vi "MS SQL_InRFID_STN10.vi"(4 "RFID":string, 5 "OP10_CRIMP":T1, 8 "error in (no error)":errorcluster, 10 "Serial No":i32, 11 "Ref in":T2={"MS SQL Connection"=refnum, "UDL File"=path "", "Time"="", "DCODE"="", "WIP+1"=0, "MC No?"=0, "POKAYOKE?"=FALSE, "Expected Result"="", "Result [Status]"="", "Clock"=0.0, "RFID"="", "WIP Queue"=refnum, "TS Parameter"={"ProfitCenterCode"="", "LineCode"="", "WorkOrderNumber"="", "Model"="", "Model_with_Prefix"="", "VendorCode"="", "SetParameterDateCode"="", "PokaYoke"=0, "Target"=1, "Live_DateCode"="", "CustomerPartNumber"="", "Hand"="", "sBarcode"=FALSE, "FCA"=0, "Ent_Stamp"=timestamp(0 s since 1904-01-01), "STS_CD"=0.0}, "Data_Queue"=[], "RFID Serial No."=""} {"TS Parameter"."FCA" format="%01d"; "TS Parameter"."Target" min=1 max=100000; "TS Parameter"."PokaYoke" min=0 max=1}) -> (0 "error out":errorcluster, 3 "Ref Out":T2={"MS SQL Connection"=refnum, "UDL File"=path "", "Time"="", "DCODE"="", "WIP+1"=0, "MC No?"=0, "POKAYOKE?"=FALSE, "Expected Result"="", "Result [Status]"="", "Clock"=0.0, "RFID"="", "WIP Queue"=refnum, "TS Parameter"={"ProfitCenterCode"="", "LineCode"="", "WorkOrderNumber"="", "Model"="", "Model_with_Prefix"="", "VendorCode"="", "SetParameterDateCode"="", "PokaYoke"=0, "Target"=1, "Live_DateCode"="", "CustomerPartNumber"="", "Hand"="", "sBarcode"=FALSE, "FCA"=0, "Ent_Stamp"=timestamp(0 s since 1904-01-01), "STS_CD"=0.0}, "Data_Queue"=[], "RFID Serial No."=""} {"TS Parameter"."FCA" format="%01d"; "TS Parameter"."Target" min=1 max=100000; "TS Parameter"."PokaYoke" min=0 max=1})   [LabVIEW 2020]
uses:
  Controls/TD SQL.ctl
  <vilib>/addons/database/Connection.llb/Conn ObjectReference.ctl
  Controls/WIP_State.ctl
  Controls/TS_Parameter.ctl
  <vilib>/addons/database/NI_Database_API.lvlib
panel:
  in  "[CT]":dbl
  in  "[STATUS]":i32
  out "resulting string":string
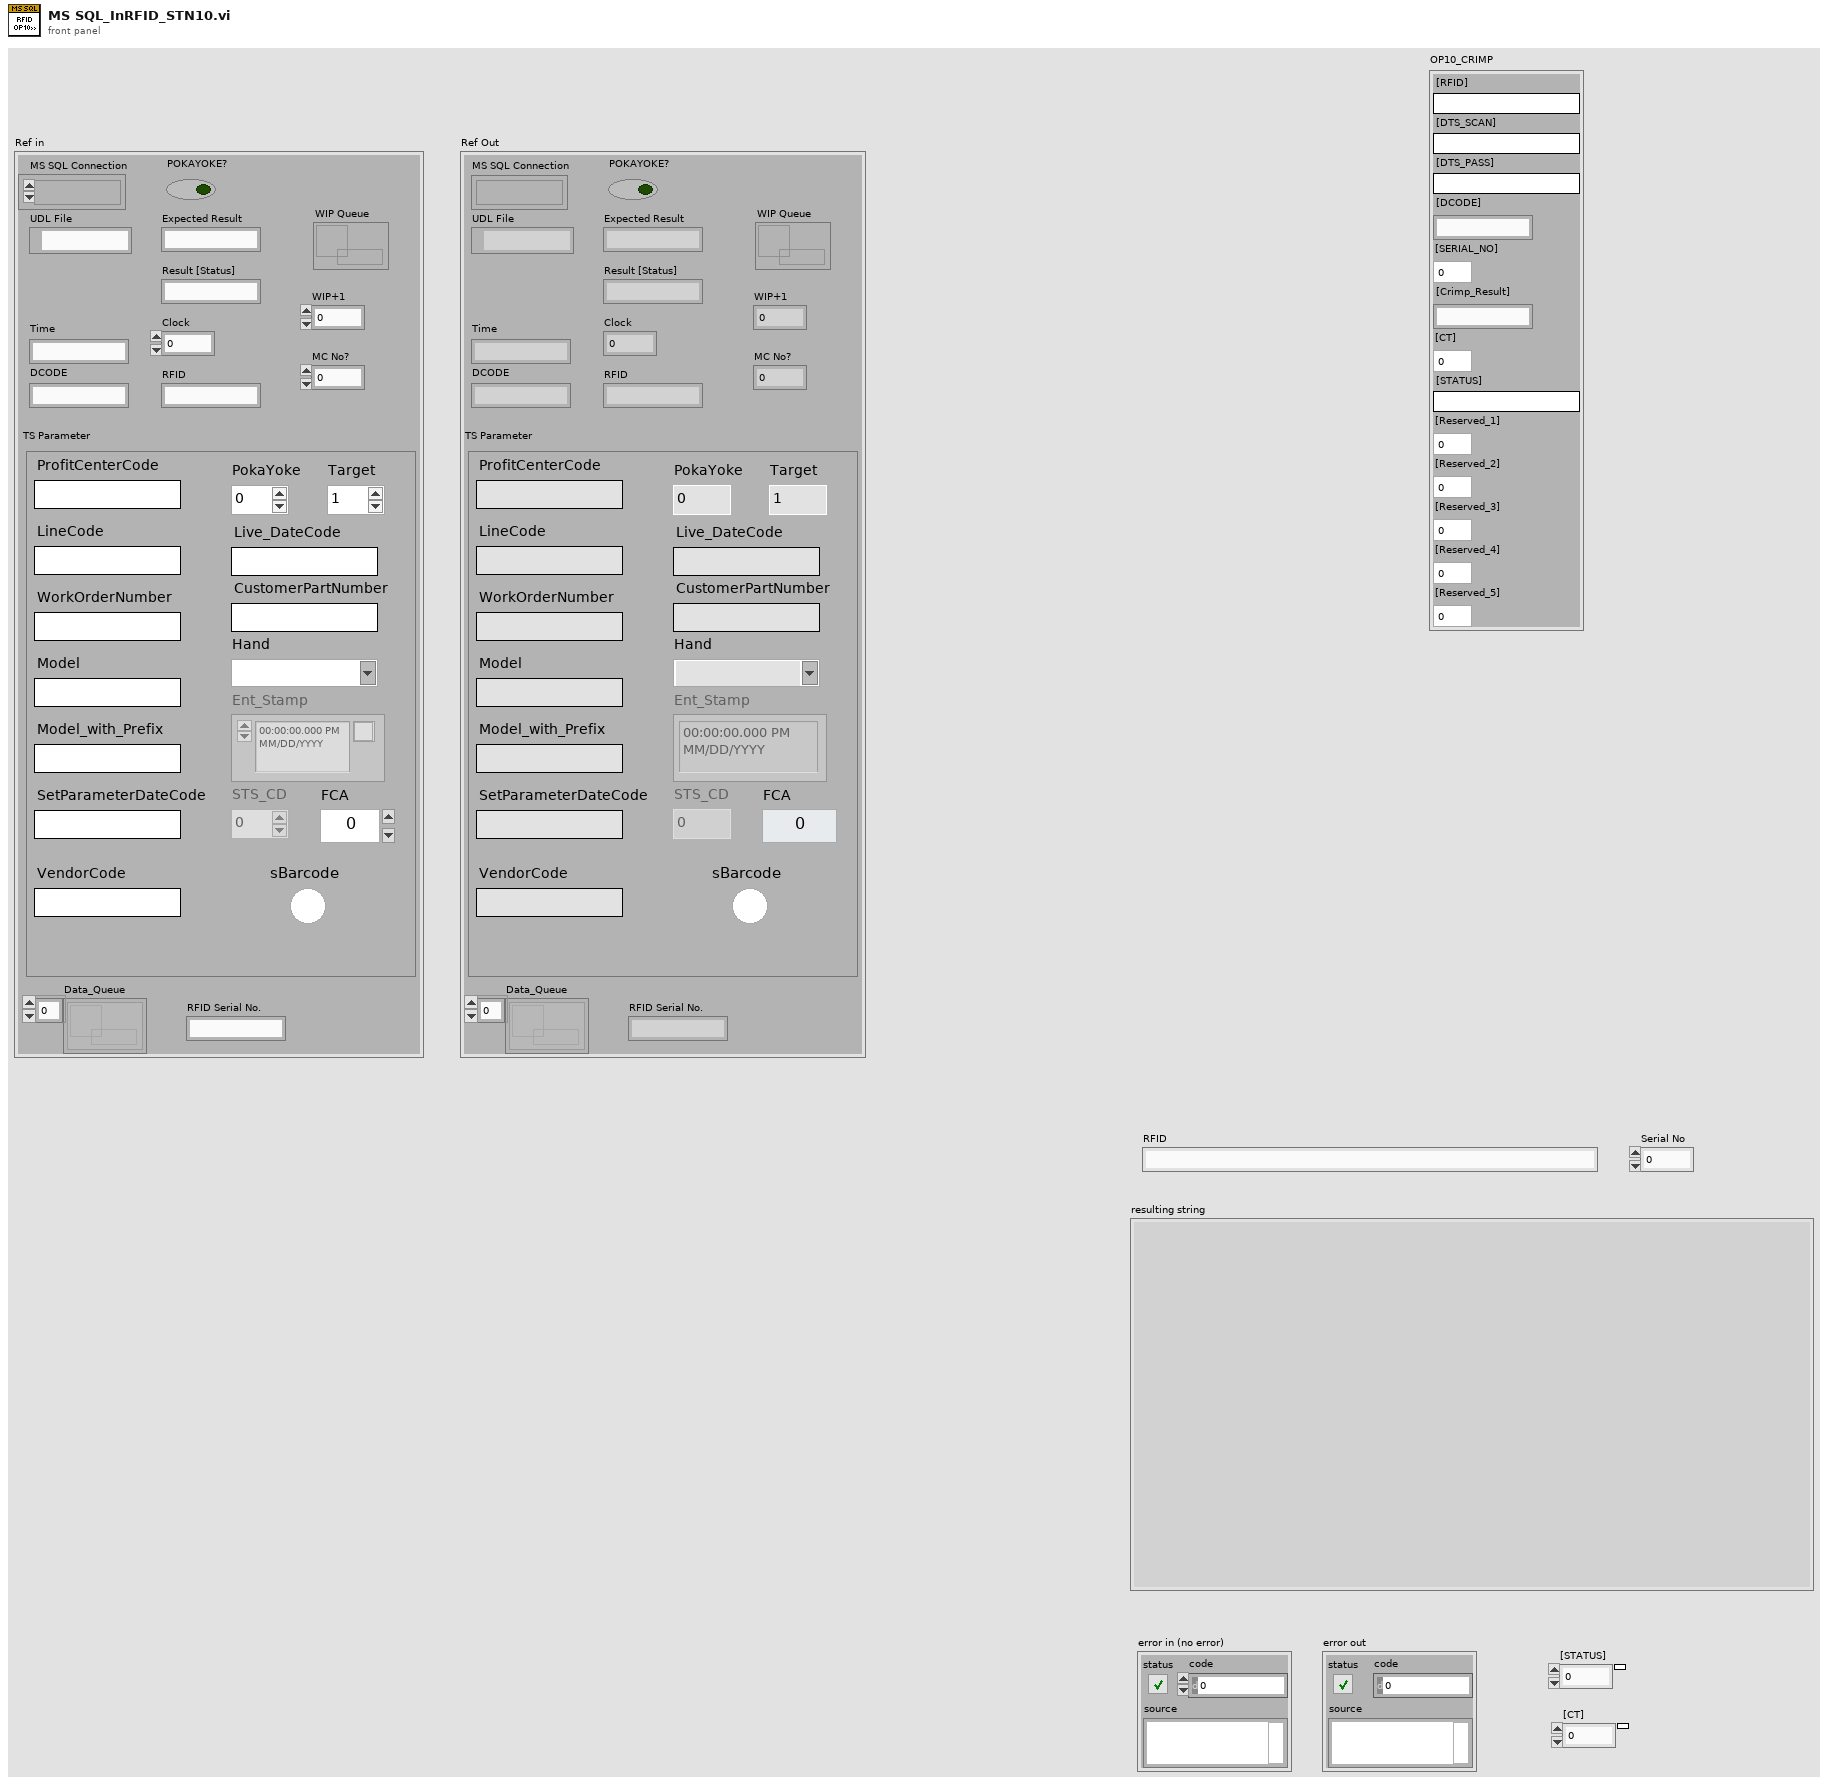
[diagram p1: front panel]
types:
  T1 = cluster{"[RFID]":string, "[DTS_SCAN]":string, "[DTS_PASS]":string, "[DCODE]":string, "[SERIAL_NO]":i32, "[Crimp_Result]":string, "[CT]":dbl, "[STATUS]":string, "[Reserved_1]":dbl, "[Reserved_2]":dbl, "[Reserved_3]":dbl, "[Reserved_4]":dbl, "[Reserved_5]":dbl}
  T2 = typedef "TD SQL.ctl" = cluster{"MS SQL Connection":T3, "UDL File":path, "Time":string, "DCODE":string, "WIP+1":i64, "MC No?":i32, "POKAYOKE?":bool, "Expected Result":string, "Result [Status]":string, "Clock":dbl, "RFID":string, "WIP Queue":refnum<queue>, "TS Parameter":T4, "Data_Queue":refnum<queue>[], "RFID Serial No.":string}
  T3 = typedef "NI_Database_API.lvlib/Conn ObjectReference.ctl" = refnum<k1>
  T4 = typedef "TS_Parameter.ctl" = cluster{"ProfitCenterCode":string, "LineCode":string, "WorkOrderNumber":string, "Model":string, "Model_with_Prefix":string, "VendorCode":string, "SetParameterDateCode":string, "PokaYoke":i32, "Target":i32, "Live_DateCode":string, "CustomerPartNumber":string, "Hand":string, "sBarcode":bool, "FCA":i32, "Ent_Stamp":timestamp, "STS_CD":dbl}
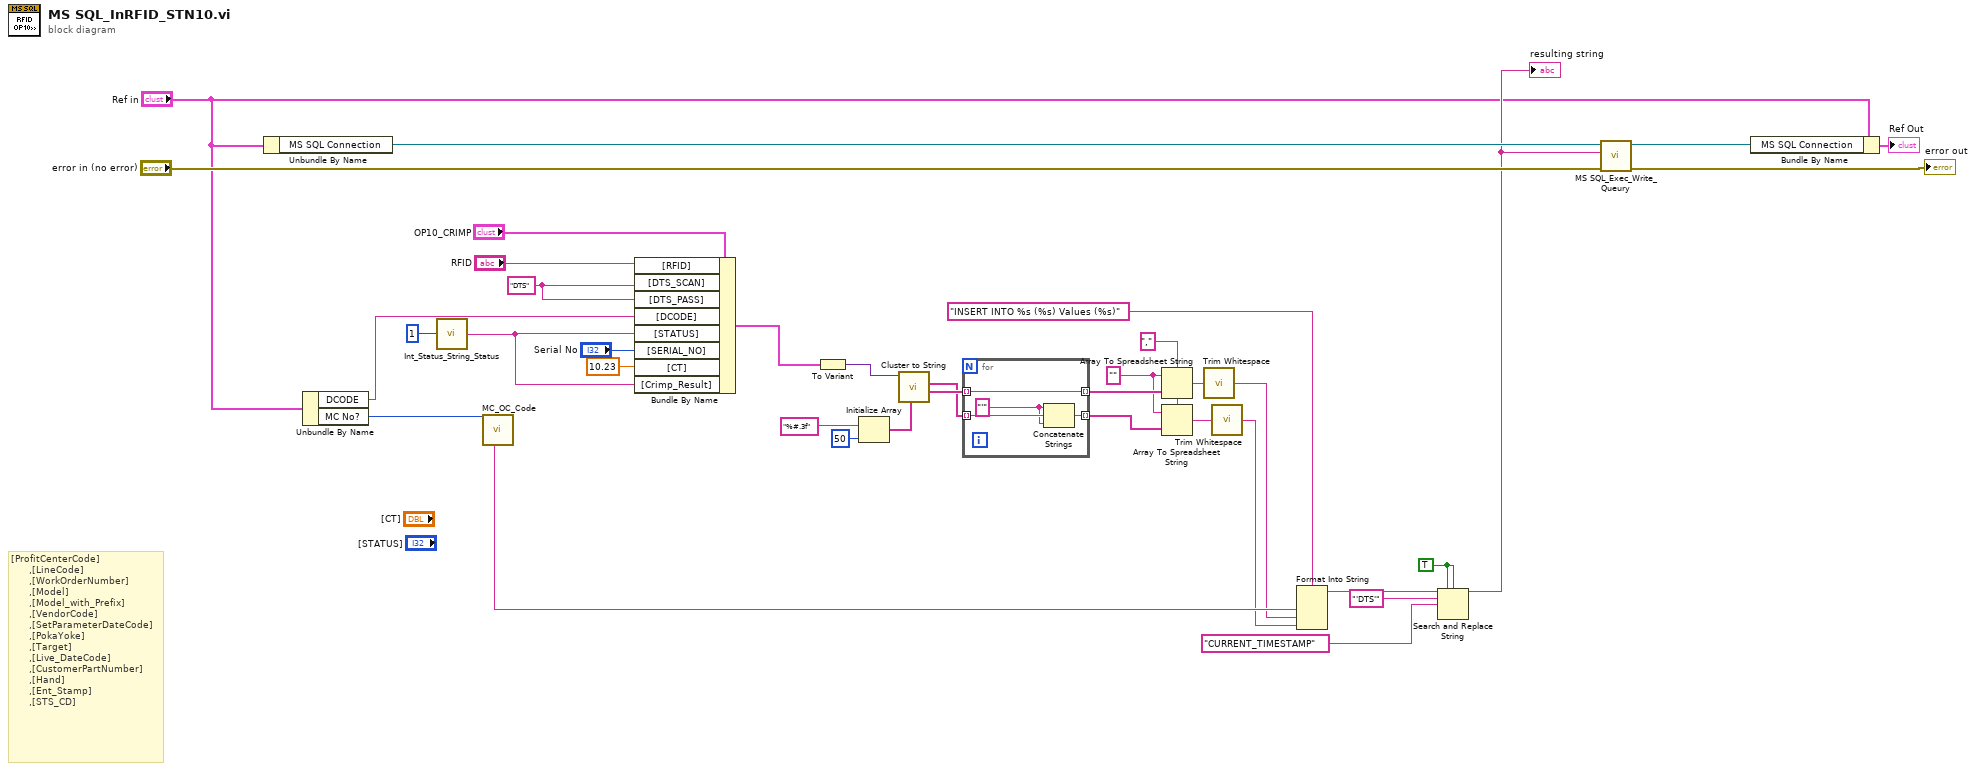
[diagram p0: block diagram]
diagram:
  w10 = TRUE ("ignore case? (F)")
  w20 = "," ("delimiter (Tab)")
  w21 = "" ("format string")
  w15 = "DTS" ("[DTS_PASS]")
  # "[ProfitCenterCode]\n      ,[LineCode]\n      ,[WorkOrderNumber]\n      ,[Model]\n      ,[Model_with_Prefix]\n      ,[VendorCode]\n      ,[SetParameterDateCode]\n      ,[PokaYoke]\n      ,[Target]\n      ,[Live_DateCode]\n      ,[CustomerPartNumber]\n      ,[Hand]\n      ,[Ent_Stamp]\n      ,[STS_CD]"
  n1 = Unbundle By Name("Ref in") -> ("MS SQL Connection"=w33:T3)
  n2 = Unbundle By Name("Ref in") -> ("DCODE"=w1:string, "MC No?"=w9:i32)
  n3 = call "Int_Status_String_Status.vi"("[STATUS]"=1) -> ("STATUS"=w3:string)
  n4 = call "MC_OC_Code.vi"("index"=w9) -> ("Table Name"=w24:string)  [unwired: 4 in, 6 out]
  n5 = Bundle By Name(cluster="OP10_CRIMP", "[RFID]"="RFID", "[DTS_SCAN]"=w15, "[DTS_PASS]"=w15, "[DCODE]"=w1, "[STATUS]"=w3, "[SERIAL_NO]"="Serial No", "[CT]"=10.23, "[Crimp_Result]"=w3) -> (w32:T1)
  n6 = To Variant(anything=w32) -> (Variant=w26:variant)
  n7 = Initialize Array("%#.3f" ("delimiter (Tab)"), 50 ("dimension size")) -> (w27:string[])
  n8 = call <userlib>:"Cluster to String.vi"("Format IN"=w27, "Variant In"=w26) -> ("Format String Name"=w30:string[], "Format String Array"=w7:string[])  [unwired: 6 in, 2 out]
  n9 = for {
    tunnel: w7 -> [w41] mode=indexing
    tunnel: [w39] -> w22 mode=indexing
    tunnel: w30 -> [w38] mode=indexing
    tunnel: [w38] -> w23 mode=indexing
    w40 = "'" ("string")
    n10 = Concatenate Strings(w40, w41, w40) -> (w39:string)
  }
  n11 = Array To Spreadsheet String(delimiter (Tab)=w20, array=w23, 3:w21) -> (spreadsheet string=w19:string)
  n12 = Array To Spreadsheet String(delimiter (Tab)=w20, array=w22, 3:w21) -> (spreadsheet string=w18:string)
  n13 = call <vilib>:"Trim Whitespace.vi"("string"=w19) -> ("trimmed string"=w17:string)  [unwired: 1 in]
  n14 = call <vilib>:"Trim Whitespace.vi"("string"=w18) -> ("trimmed string"=w16:string)  [unwired: 1 in]
  n15 = Format Into String(format string="INSERT INTO %s (%s) Values (%s)" ("delimiter (Tab)"), w24, w17, w16) -> (resulting string=w14:string)  [unwired: 2 in, 1 out]
  n16 = Search and Replace String(replace all?=w10, case sensitive?=w10, input string=w14, search string="'DTS'" ("delimiter (Tab)"), replace string="CURRENT_TIMESTAMP" ("delimiter (Tab)")) -> (result string=w13:string)  [unwired: 3 in, 3 out]
  "resulting string" <- w13
  n17 = call "MS SQL_Exec_Write_Queury.vi"("error in (no error)"="error in (no error)", "Query"=w13, "Refnum in"=w33) -> ("error out"=→"error out":errorcluster, "Refnum out"=w35:T3)  [unwired: 7 in]
  n18 = Bundle By Name(cluster="Ref in", "MS SQL Connection"=w35) -> (→"Ref Out":T2)
